vi "Online Save Status.vi"(8 "error in (no error)":errorcluster, 9 "SN":string, 10 "Complete":bool, 11 "Status":bool) -> (0 "error out":errorcluster, 3 "information":T1)   [LabVIEW 2014]
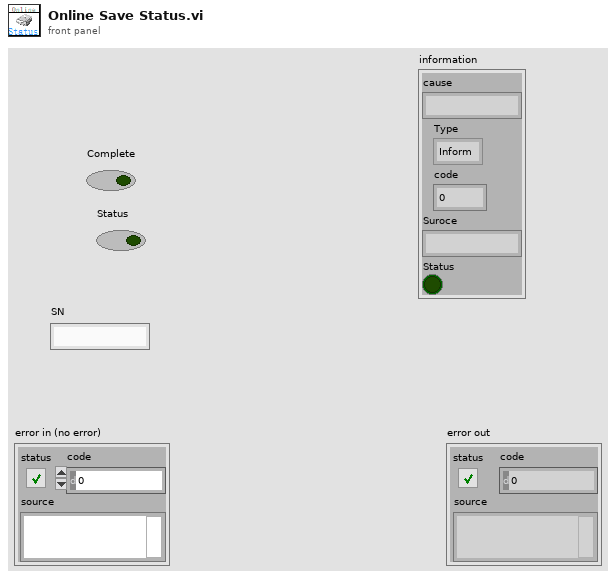
[diagram p1: front panel]
types:
  T1 = cluster{"cause":string, "Type":enum16{"Inform", "Warning", "Alarm"}, "code":i32, "Suroce":string, "Status":bool}
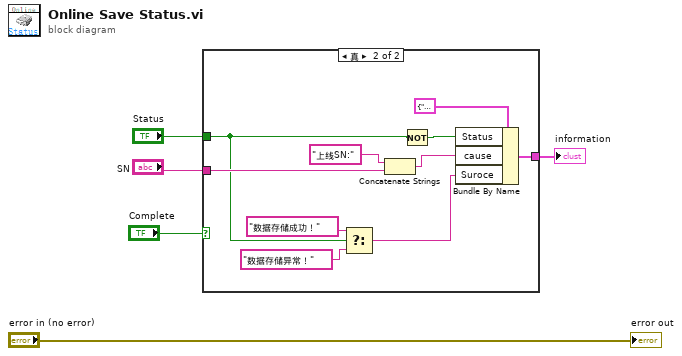
[diagram p0: block diagram]
diagram:
  n1 = case shown="真" "Complete" {
    tunnel: "Status" -> [_ w8]
    tunnel: "SN" -> [_ w13]
    tunnel: [_ w11] -> w2
    frame False {
    }
    frame True {
      n2 = Select(t="数据存储成功！", s=w8, f="数据存储异常！") -> (s? t:f=w6:string)
      n3 = Concatenate Strings("上线SN:", w13) -> (w12:string)
      n4 = Not(x=w8) -> (.not. x?=w9:bool)
      n5 = Bundle By Name(cluster=T1 {"cause"="", "Type"=enum."Inform", "code"=0, "Suroce"="", "Status"=FALSE} ("information"), "Status"=w9, "cause"=w12, "Suroce"=w6) -> (w11:T1)
    }
  }
  "information" <- w2
  "error out" <- "error in (no error)"
